vi "formato_aquisicao_global_adq.vi"() -> ()   [LabVIEW 2019]
panel:
  in  "NATIONAL/\nWIRELESS":bool
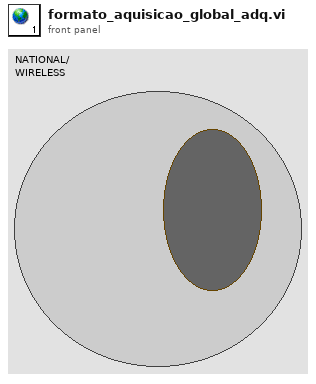
[diagram p1: front panel]
diagram:
